vi "releaseQueues.vi"(8 "error in (no error)":errorcluster, 11 "TcpServerBase in":refnum<class "TcpServerBase.lvclass">) -> (0 "error out":errorcluster, 3 "TcpServerBase out":refnum<class "TcpServerBase.lvclass">)   [LabVIEW 2018, in "TcpServerBase.lvclass"]
doc: "Release queueServerCmd, queueServerTel, queueClientCmd, queueClientTel, queueStateMachineCmd, and queueStateMachineTel."
uses:
  TcpServerBase.lvclass
  TcpServerBase.lvclass/TcpServerBase.ctl
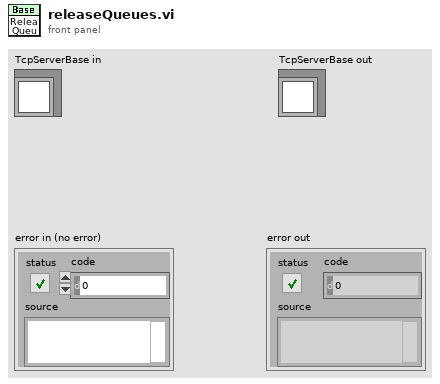
[diagram p1: front panel]
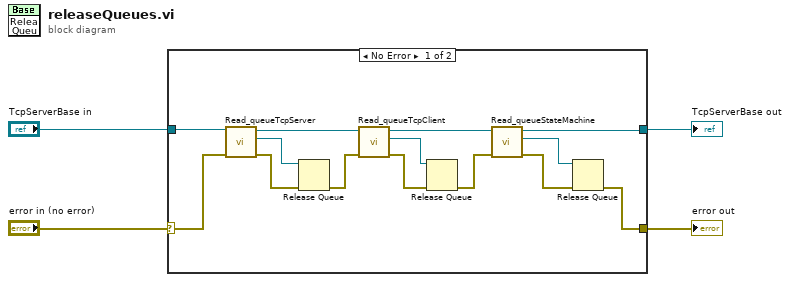
[diagram p0: block diagram]
diagram:
  n1 = case shown="No Error" "error in (no error)" {
    selector: "error in (no error)" -> [w13 w19]
    tunnel: "TcpServerBase in" -> [w14 w20]
    tunnel: [w6 w20] -> w2
    tunnel: [w5 w19] -> w1
    frame No Error {
      n2 = call "Read_queueTcpServer.vi"("error in (no error)"=w13, "TcpServerBase in"=w14) -> ("error out"=w15:errorcluster, "queueTcpServer"=w16:refnum<queue>, "TcpServerBase out"=w12:refnum<class "TcpServerBase.lvclass">)  [unwired: 7 in]
      n3 = Release Queue(queue=w16, error in (no error)=w15) -> (error out=w10:errorcluster)  [unwired: 1 in, 2 out]
      n4 = call "Read_queueTcpClient.vi"("error in (no error)"=w10, "TcpServerBase in"=w12) -> ("error out"=w9:errorcluster, "queueTcpClient"=w8:refnum<queue>, "TcpServerBase out"=w11:refnum<class "TcpServerBase.lvclass">)  [unwired: 7 in]
      n5 = Release Queue(queue=w8, error in (no error)=w9) -> (error out=w7:errorcluster)  [unwired: 1 in, 2 out]
      n6 = call "Read_queueStateMachine.vi"("error in (no error)"=w7, "TcpServerBase in"=w11) -> ("error out"=w18:errorcluster, "queueStateMachine"=w17:refnum<queue>, "TcpServerBase out"=w6:refnum<class "TcpServerBase.lvclass">)  [unwired: 7 in]
      n7 = Release Queue(queue=w17, error in (no error)=w18) -> (error out=w5:errorcluster)  [unwired: 1 in, 2 out]
    }
    frame Error {
    }
  }
  "error out" <- w1
  "TcpServerBase out" <- w2
